vi "create EIP channel.vi"(5 "output?":bool, 7 "element index":i32, 8 "eip tag type":T1, 9 "Tag Name":string, 10 "Network Path":string, 11 "name":string) -> (3 "EthernetIP Channel out":refnum<class "EIP Tags Channel.lvclass">)   [LabVIEW 2013, in "EIP Tags Channel.lvclass"]
uses:
  EIP Tags Channel.lvclass
  configuration/eip tag types.ctl
  <vilib>/NI/Tag Bus Module Framework/channel/channel classification.ctl
  <vilib>/NI/Tag Bus/tag/tag descriptor.lvclass/tag descriptor.ctl
  <vilib>/NI/Tag Bus Module Framework/channel/TBM channel.lvclass/TBM channel.ctl
  EIP Tags Channel.lvclass/EIP Tags Channel.ctl
  <vilib>/NI/Tag Bus/tag/tag descriptor.lvclass
  <vilib>/NI/Tag Bus Module Framework/channel/TBM channel.lvclass
  configuration/EIP Tags Configuration.lvclass
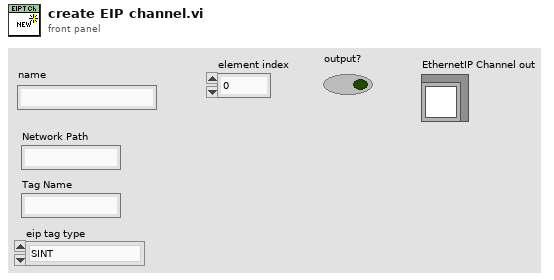
[diagram p1: front panel]
types:
  T1 = typedef "EIP Tags Configuration.lvclass/eip tag types.ctl" = enum16{"SINT", "INT", "DINT", "REAL", "BOOL", "STRING"}
  T2 = typedef "TBM channel.lvclass/channel classification.ctl" = enum16{"input data", "output data", "processing parameter", "processing result"}
  T3 = typedef "tag bus.lvlib/tag descriptor.lvclass/Data Type.ctl" = enum16{"Double", "Single", "I64", "I32", "I16", "I8", "U64", "U32", "U16", "U8", "Boolean", "String", "Array of Double", "Array of Single", "Array of I64", "Array of I32", "Array of I16", "Array of I8", "Array of U64", "Array of U32", "Array of U16", "Array of U8", "Array of Boolean", "Array of String"}
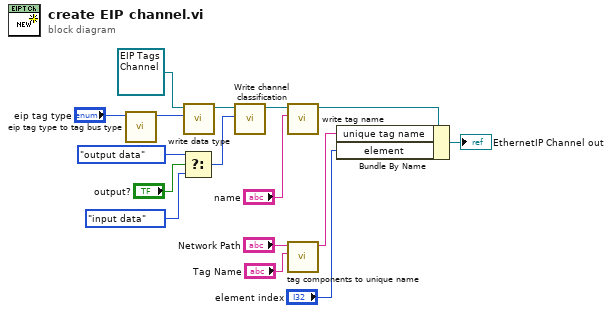
[diagram p0: block diagram]
diagram:
  n1 = call "eip tag type to tag bus type.vi"("eip tag types"="eip tag type") -> ("data type"=w10:T3)  [unwired: 10 in]
  n2 = Select(t=channel_classification."output data" ("channel classification"), s="output?", f=channel_classification."input data" ("channel classification")) -> (s? t:f=w5:T2)
  n3 = call <vilib>:"write data type.vi"("data type"=w10, "system tag in"=refnum<class "EIP Tags Channel.lvclass"> refnum ("EthernetIP Channel in")) -> ("system tag out"=w14:refnum<class "EIP Tags Channel.lvclass">)  [unwired: 8 in, 1 out]
  n4 = call <vilib>:"Write channel classification.vi"("channel classification"=w5, "channel in"=w14) -> ("channel out"=w11:refnum<class "EIP Tags Channel.lvclass">)  [unwired: 8 in, 1 out]
  n5 = call <vilib>:"write tag name.vi"("name"="name", "system tag in"=w11) -> ("system tag out"=w15:refnum<class "EIP Tags Channel.lvclass">)  [unwired: 8 in, 1 out]
  n6 = call "tag components to unique name.vi"("Tag Name"="Tag Name", "Network Path"="Network Path") -> ("unique name"=w1:string)  [unwired: 9 in]
  n7 = Bundle By Name(cluster=w15, "unique tag name"=w1, "element"="element index") -> (→"EthernetIP Channel out":refnum<class "EIP Tags Channel.lvclass">)
